vi "Enable Bus Display.vi"(8 "error in (no error)":errorcluster, 9 "Enable Bus Display (T: Enable)":bool=TRUE, 10 "Bus Name (1: Digital Bus 1)":i32(ring)=1 items=["Digital Bus 1"=1, "Digital Bus 2"=2], 11 "VISA resource name":refnum<visa-resource-name>) -> (0 "error out":errorcluster, 3 "VISA resource name out":refnum<visa-resource-name>)   [LabVIEW 2015, in "Agilent 2000 3000 X-Series.lvlib"]
doc: "Configures the digital bus display.\n\n<B>Note(s)</B>\nThis operation is only valid for the MSO models."
uses:
  Agilent 2000 3000 X-Series.lvlib
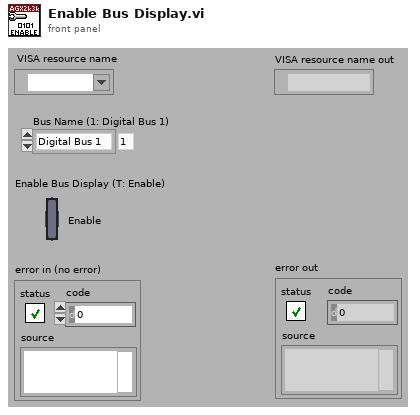
[diagram p1: front panel]
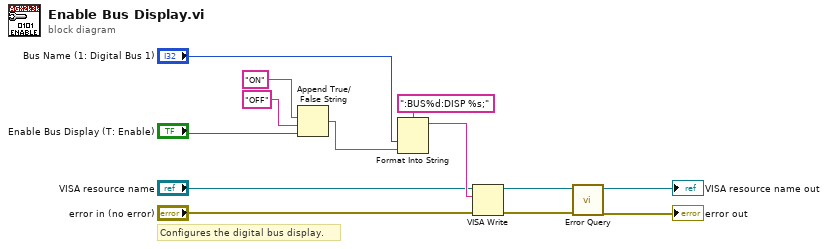
[diagram p0: block diagram]
diagram:
  # "Configures the digital bus display."
  n1 = Append True/False String(1:"Enable Bus Display (T: Enable)", 2:"OFF", 3:"ON") -> (0:w9:string)  [unwired: 1 out]
  n2 = Format Into String(format string=":BUS%d:DISP %s;", "Bus Name (1: Digital Bus 1)", w9) -> (resulting string=w8:string)  [unwired: 2 in, 1 out]
  n3 = VISA Write(VISA resource name="VISA resource name", write buffer=w8, error in (no error)="error in (no error)") -> (VISA resource name out=w5:refnum<visa-resource-name>, error out=w4:errorcluster)  [unwired: 1 out]
  n4 = call "Error Query.vi"("error in (no error)"=w4, "VISA resource name"=w5) -> ("error out"=→"error out":errorcluster, "VISA resource name out"=→"VISA resource name out":refnum<visa-resource-name>)  [unwired: 8 out]
